vi "Configure Peak Search Sort.vi"(0 "VISA resource name":refnum<visa-resource-name>, 5 "Sort Mode (0:Sort X)":i32(ring) items=["Sort X", "Sort Y", "Set Number"], 7 "Number (10)":i32=10 min=1 max=10, 11 "error in (no error)":errorcluster) -> (4 "VISA resource name out":refnum<visa-resource-name>, 15 "error out":errorcluster)   [LabVIEW 2020, in "Anritsu Signal Analyzer Series.lvlib"]
doc: "Configures the Marker Search Peaks sort settings of the spectrum analyzer."
uses:
  Anritsu Signal Analyzer Series.lvlib
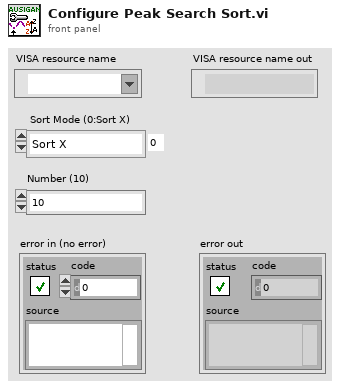
[diagram p1: front panel]
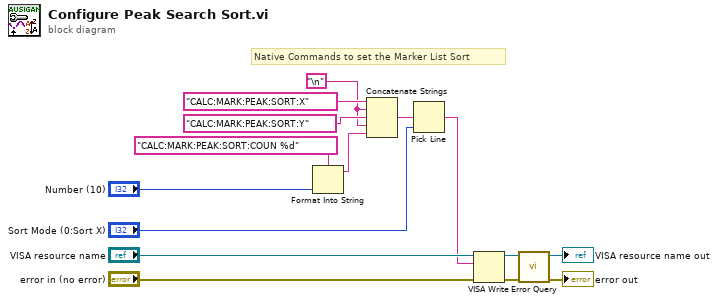
[diagram p0: block diagram]
diagram:
  w5 = "\n"
  # "Native Commands to set the Marker List Sort"
  n1 = Format Into String(format string="CALC:MARK:PEAK:SORT:COUN %d" ("Format String"), "Number (10)") -> (resulting string=w3:string)  [unwired: 2 in, 1 out]
  n2 = Concatenate Strings("CALC:MARK:PEAK:SORT:X" ("_Command"), w5, "CALC:MARK:PEAK:SORT:Y" ("_Command"), w5, w3) -> (w2:string)
  n3 = Pick Line(multi-line string=w2, line index="Sort Mode (0:Sort X)") -> (output string=w1:string)  [unwired: 1 in]
  n4 = VISA Write(VISA resource name="VISA resource name", write buffer=w1, error in (no error)="error in (no error)") -> (VISA resource name out=w8:refnum<visa-resource-name>, error out=w9:errorcluster)  [unwired: 1 out]
  n5 = call "Error Query.vi"("error in (no error)"=w9, "VISA resource name"=w8) -> ("error out"=→"error out":errorcluster, "VISA resource name out"=→"VISA resource name out":refnum<visa-resource-name>)  [unwired: 6 in, 2 out]
